vi "utility.SCI.Comunication.Check.vi"(7 "baud rate (9600)":u32=38400 caption="波特率(9600)", 8 "error in (no error)":errorcluster caption="错误输入（无错误）", 9 "Write":string="AA", 10 "flow control (0:none)":u16(ring)=2 caption="流控制（0:无）" items=["无", "XON/XOFF", "RTS/CTS", "XON/XOFF & RTS/CTS", "DTR/DSR", "XON/XOFF & DTR/DSR"], 11 "VISA resource name":refnum<visa-resource-name>="COM4" caption="VISA资源名称") -> (0 "错误输出":errorcluster, 1 "Output":string)   [LabVIEW 2012, in "Lib_UEL.ATE.lvlib" / "Lib_App.lvlib"]
uses:
  <vilib>/Instr/_visa.llb/VISA Configure Serial Port (Instr).vi
  Lib_App.lvlib
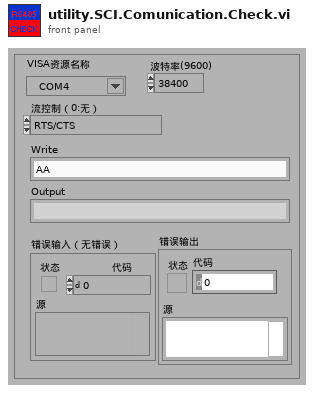
[diagram p1: front panel]
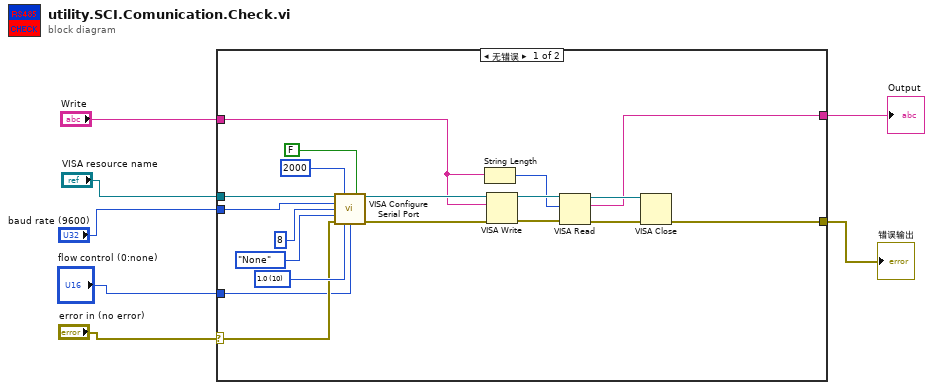
[diagram p0: block diagram]
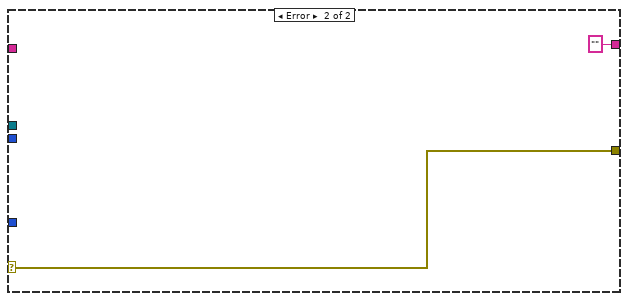
[diagram p2: hidden frame]
diagram:
  n1 = case shown="无错误" "error in (no error)" {
    selector: "error in (no error)" -> [w18 w28]
    tunnel: "VISA resource name" -> [w19 _]
    tunnel: "baud rate (9600)" -> [w16 _]
    tunnel: "flow control (0:none)" -> [w15 _]
    tunnel: "Write" -> [w11 _]
    tunnel: [w12 w28] -> w2
    tunnel: [w9 "" ("read buffer")] -> w1
    frame No Error {
      w22 = u16 10 items=["1.0"=10, "1.5"=15, "2.0"=20] ("stop bits (10: 1 bit)")
      n2 = call-poly "VISA Configure Serial Port"("VISA resource name"=w19, "timeout (10sec)"=u32 2000, "Enable Termination\nChar (T)"=FALSE ("Enable Termination\nChar (T)"), "baud rate (9600)"=w16, "data bits (8)"=u16 8, "parity (0:none)"=enum16{"None", "Odd", "Even", "Mark", "Space"}."None", "error in (no error)"=w18, "stop bits (10: 1 bit)"=w22, "flow control (0:none)"=w15) -> ("VISA resource name out"=w20:refnum<visa-resource-name>, "error out"=w21:errorcluster)  [unwired: 5 in]
      n3 = String Length(string=w11) -> (length=w10:i32)
      n4 = VISA Write(VISA resource name=w20, write buffer=w11, error in (no error)=w21) -> (VISA resource name out=w26:refnum<visa-resource-name>, error out=w25:errorcluster)  [unwired: 1 out]
      n5 = VISA Read(VISA resource name=w26, byte count=w10, error in (no error)=w25) -> (VISA resource name out=w14:refnum<visa-resource-name>, read buffer=w9:string, error out=w13:errorcluster)  [unwired: 1 out]
      n6 = VISA Close(VISA resource name=w14, error in (no error)=w13) -> (error out=w12:errorcluster)
    }
    frame Error {
    }
  }
  "错误输出" <- w2
  "Output" <- w1
